vi "SerialRead.vi"() -> ()   [LabVIEW 2013]
uses:
  <vilib>/Analysis/3filter.llb/Filter Passband Type.ctl
  <vilib>/Instr/_visa.llb/VISA Configure Serial Port (Instr).vi
  <vilib>/Analysis/3filter.llb/Butterworth Filter (DBL).vi
  <vilib>/Analysis/NI_AALBase.lvlib
panel:
  in  "?":bool
  out "time":dbl
  in  "high_time":i32
  in  "low_time":i32
  out "diferença":dbl
  out "high_time":dbl format="%#_10g"
  out "low_time":dbl format="%#_10g"
  in  "stop":bool
  in  "high":u32
  in  "low":i32
  in  "Pcell1":u32[](array[numeric])
  in  "Pcell2":u32[](array[numeric])
  in  "Pcell3":u32[](array[numeric])
  in  "Pcell4":u32[](array[numeric])
  in  "cell1":u32[](array[numeric])
  in  "cell2":u32[](array[numeric])
  in  "cell3":u32[](array[numeric])
  in  "cell4":u32[](array[numeric])
  in  "last":u32
  out "time":u32[](graph)
  in  "Tab Control":enum32{"raw data", "filter", "weight"}(tab)
  out "filter_cell2":dbl[](graph) caption="Sine"
  out "filter_cell4":dbl[](graph) caption="Sine"
  out "filter_cell3":dbl[](graph) caption="Sine"
  out "filter_cell1":dbl[](graph) caption="Sine"
  out "peso_cell2":dbl[](graph) caption="Sine"
  out "peso_cell3":dbl[](graph) caption="Sine"
  out "peso_cell4":dbl[](graph) caption="Sine"
  out "peso_cell1":dbl[](graph) caption="Sine"
  out "cell":u8[](array[numeric])
  out "output_int16":i32[](array[numeric])
  out "data":u8[](array[numeric])
  in  "serial_port":refnum<visa-resource-name> caption="Porta Serial"
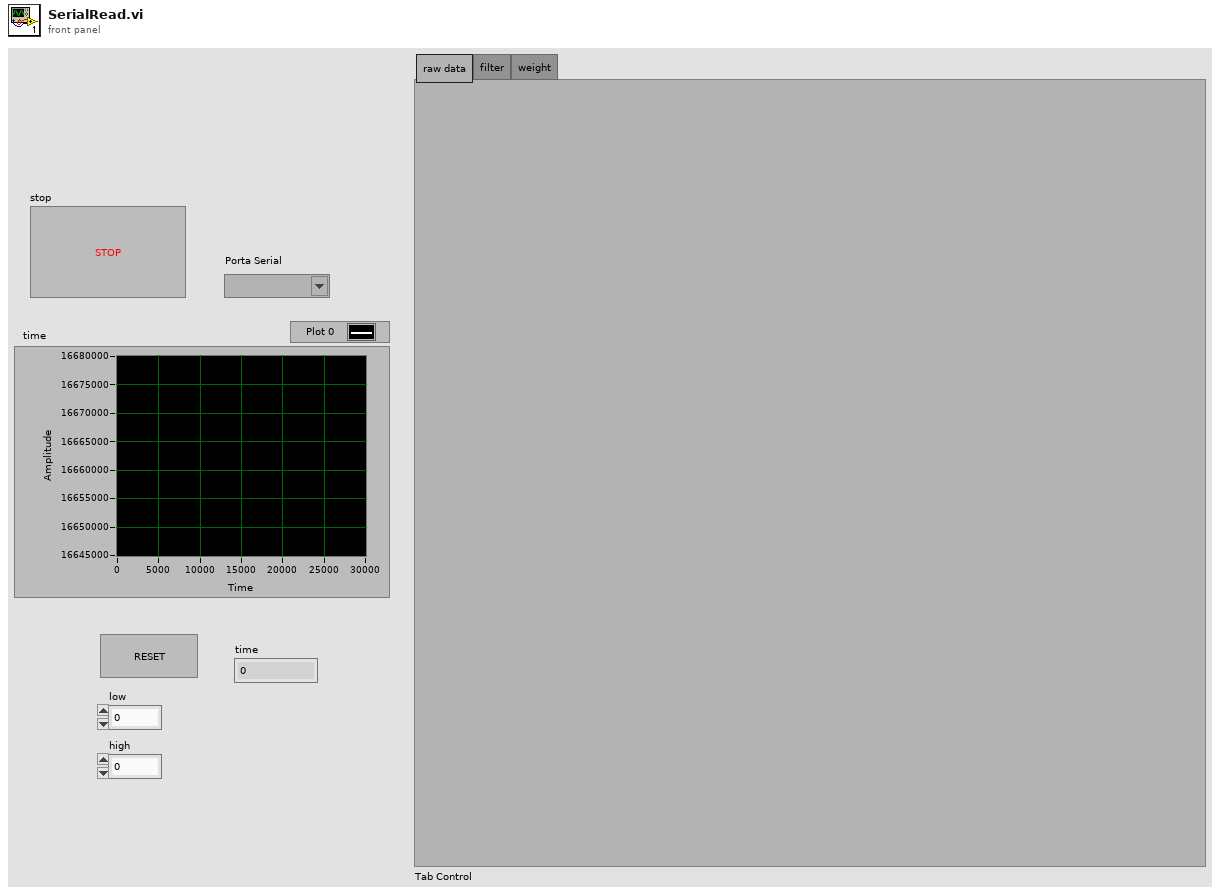
[diagram p1: front panel]
types:
  T1 = typedef "NI_AALBase.lvlib/Filter Passband Type.ctl" = enum32{"Lowpass", "Highpass", "Bandpass", "Bandstop"}
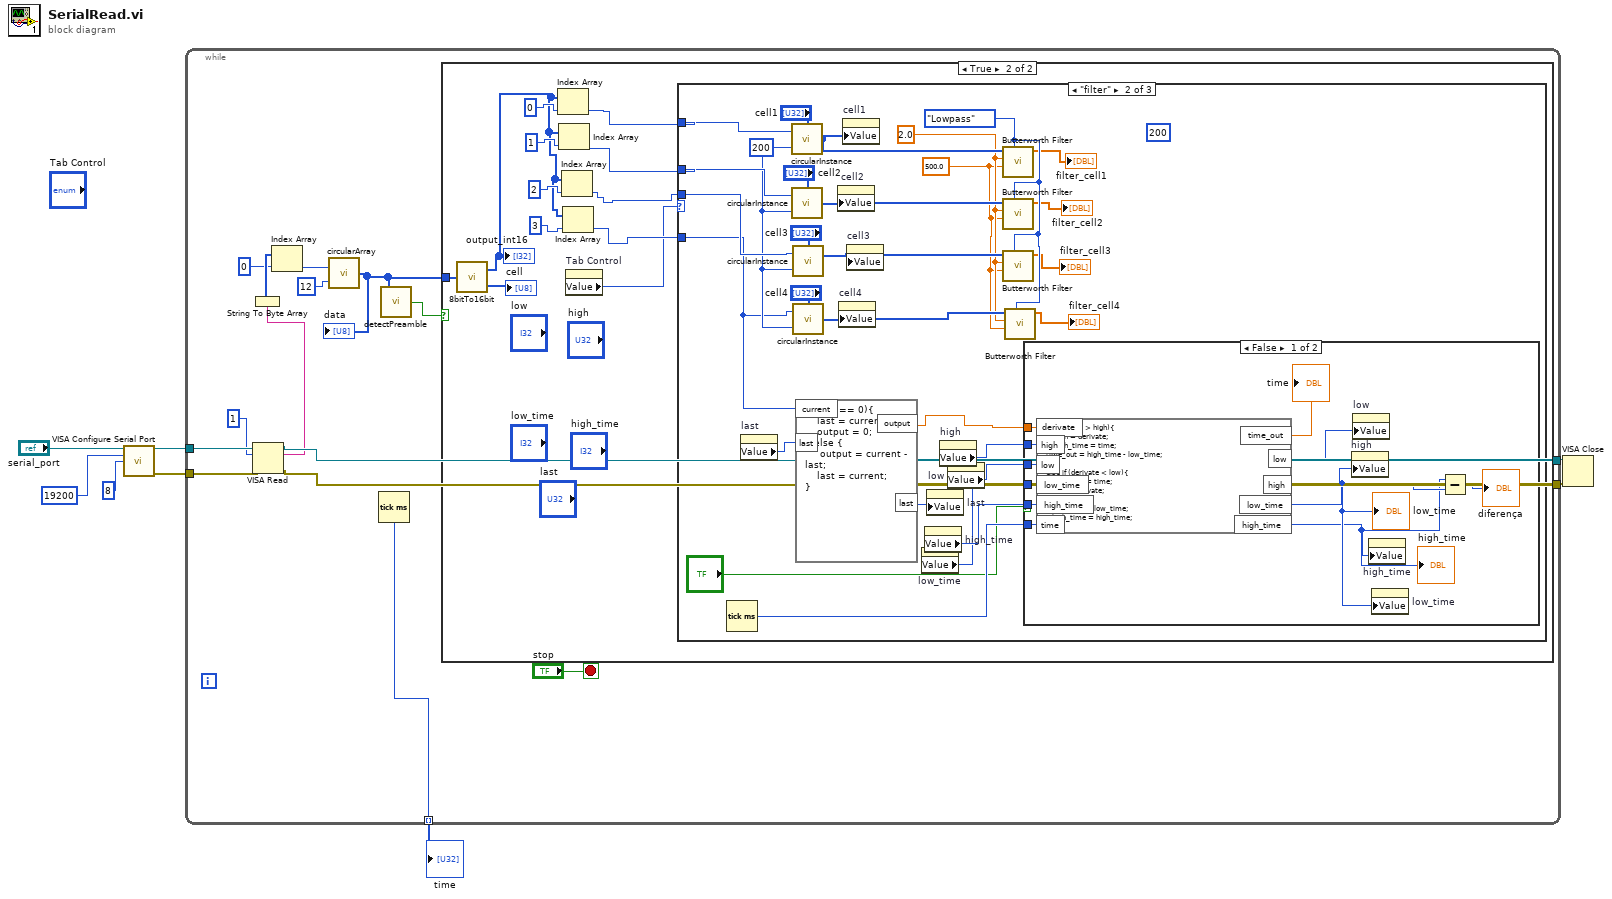
[diagram p0: block diagram]
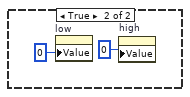
[diagram p4: hidden frame]
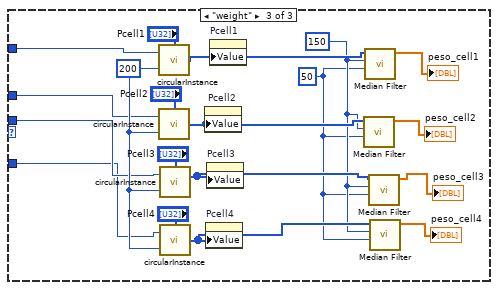
[diagram p5: hidden frame]
diagram:
  n1 = call-poly "VISA Configure Serial Port"("VISA resource name"="serial_port", "baud rate (9600)"=u32 19200, "data bits (8)"=u16 8) -> ("VISA resource name out"=w5:refnum<visa-resource-name>, "error out"=w4:errorcluster)  [unwired: 11 in]
  n2 = while {
    tunnel: w5 -> [w22]
    tunnel: w4 -> [w21]
    tunnel: [w19] -> w2
    tunnel: [w20] -> w3
    tunnel: [w10] -> w1 mode=indexing
    stop <- "stop" stop-if-true
    n3 = VISA Read(VISA resource name=w22, byte count=1, error in (no error)=w21) -> (VISA resource name out=w20:refnum<visa-resource-name>, read buffer=w14:string, error out=w19:errorcluster)  [unwired: 1 out]
    n4 = String To Byte Array(string=w14) -> (unsigned byte array=w17:u8[])
    n5 = Index Array(array=w17, index=0) -> (element=w11:u8)
    n6 = call "circularArray.vi"("max-size"=u8 12, "element"=w11) -> ("dataout"=w12:u8[])
    "data" <- w12
    n7 = Tick Count (ms)() -> (millisecond timer value=w10:u32)
    n8 = call "detectPreamble.vi"("data-in"=w12) -> ("detected"=w9:bool)
    n9 = case shown="True" w9 {
      tunnel: w12 -> [_ w33]
      frame False {
      }
      frame True {
        n10 = call "8bitTo16bit.vi"("input_byte"=w33) -> ("output_int16"=w28:i32[], "cell"=→"cell":u8[])
        "output_int16" <- w28
        n11 = Index Array(array=w28, index=0) -> (element=w24:i32)
        n12 = Index Array(array=w28, index=1) -> (element=w25:i32)
        n13 = Index Array(array=w28, index=2) -> (element=w26:i32)
        n14 = Index Array(array=w28, index=3) -> (element=w27:i32)
        n15 = property on="Tab Control" class="TabCtl (strict)"() -> ("Value"=w23:enum32{"raw data", "filter", "weight"})  [unwired: 2 in, 2 out]
        n16 = case shown="\"filter\"" w23 {
          tunnel: w24 -> [_ w63 w91]
          tunnel: w25 -> [_ w62 w90]
          tunnel: w26 -> [_ w57 w89]
          tunnel: w27 -> [_ w44 w88]
          frame "raw data", Default {
          }
          frame "filter" {
            (unwired) 200
            w52 = 2.0 ("sampling freq: fs")
            w51 = 500.0 ("high cutoff freq: fh")
            w50 = Filter_Passband_Type."Lowpass" ("filter type")
            w46 = i16 200 ("max-size")
            n17 = Tick Count (ms)() -> (millisecond timer value=w37:u32)
            n18 = property on="last" class="DigNum (strict)"() -> ("Value"=w45:u32)  [unwired: 2 in, 2 out]
            n19 = call "circularInstance.vi"("data"="cell1", "max-size"=w46, "element"=w63) -> ("dataout"=w58:u32[])
            n20 = call "circularInstance.vi"("data"="cell2", "max-size"=w46, "element"=w62) -> ("dataout"=w59:u32[])
            n21 = call "circularInstance.vi"("data"="cell3", "max-size"=w46, "element"=w57) -> ("dataout"=w55:u32[])
            n22 = call "circularInstance.vi"("data"="cell4", "max-size"=w46, "element"=w44) -> ("dataout"=w53:u32[])
            n23 = formula code="if (last == 0){\n    last = current;\n    output = 0;\n} else {\n     output = current - last;\n    last = current;\n}"("last"=w45, "current"=w44) -> ("output"=w42:dbl, "last"=w43:u32)
            n24 = property on="cell2" class="Arr (strict)"("Value"=w59) -> ()  [unwired: 2 in, 2 out]
            n25 = property on="cell4" class="Arr (strict)"("Value"=w53) -> ()  [unwired: 2 in, 2 out]
            n26 = property on="cell1" class="Arr (strict)"("Value"=w58) -> ()  [unwired: 2 in, 2 out]
            n27 = property on="cell3" class="Arr (strict)"("Value"=w55) -> ()  [unwired: 2 in, 2 out]
            n28 = property on="low_time" class="DigNum (strict)"() -> ("Value"=w38:i32)  [unwired: 2 in, 2 out]
            n29 = property on="high_time" class="DigNum (strict)"() -> ("Value"=w39:i32)  [unwired: 2 in, 2 out]
            n30 = property on="last" class="DigNum (strict)"("Value"=w43) -> ()  [unwired: 2 in, 2 out]
            n31 = property on="high" class="DigNum (strict)"() -> ("Value"=w41:u32)  [unwired: 2 in, 2 out]
            n32 = property on="low" class="DigNum (strict)"() -> ("Value"=w40:i32)  [unwired: 2 in, 2 out]
            n33 = call-poly <vilib>:"Butterworth Filter.vi"("filter type"=w50, "high cutoff freq: fh"=w51, "sampling freq: fs"=w52, "X"=w58) -> ("Filtered X"=→"filter_cell1":dbl[])  [unwired: 4 in, 1 out]
            n34 = call-poly <vilib>:"Butterworth Filter.vi"("filter type"=w50, "high cutoff freq: fh"=w51, "sampling freq: fs"=w52, "X"=w59) -> ("Filtered X"=→"filter_cell2":dbl[])  [unwired: 4 in, 1 out]
            n35 = call-poly <vilib>:"Butterworth Filter.vi"("filter type"=w50, "high cutoff freq: fh"=w51, "sampling freq: fs"=w52, "X"=w55) -> ("Filtered X"=→"filter_cell3":dbl[])  [unwired: 4 in, 1 out]
            n36 = call-poly <vilib>:"Butterworth Filter.vi"("filter type"=w50, "high cutoff freq: fh"=w51, "sampling freq: fs"=w52, "X"=w53) -> ("Filtered X"=→"filter_cell4":dbl[])  [unwired: 4 in, 1 out]
            n37 = case shown="False" "?" {
              tunnel: w42 -> [w75 _]
              tunnel: w41 -> [w74 _]
              tunnel: w40 -> [w73 _]
              tunnel: w39 -> [w69 _]
              tunnel: w38 -> [w68 _]
              tunnel: w37 -> [w65 _]
              frame False {
                n38 = formula code="if (derivate > high){\n    high = derivate;\n    high_time = time;\ntime_out = high_time - low_time;\n}\nelse if (derivate < low){\n   low_time = time;\n   low = derivate;  \n} else {\n   low_time = low_time;\n   high_time = high_time;\n}"("derivate"=w75, "high"=w74, "low"=w73, "time"=w65, "low_time"=w68, "high_time"=w69) -> ("low"=w72:i32, "high"=w71:u32, "low_time"=w67:i32, "high_time"=w66:i32, "time_out"=→"time":dbl)
                "low_time" <- w67
                "high_time" <- w66
                n39 = property on="high" class="DigNum (strict)"("Value"=w71) -> ()  [unwired: 2 in, 2 out]
                n40 = property on="low" class="DigNum (strict)"("Value"=w72) -> ()  [unwired: 2 in, 2 out]
                n41 = property on="high_time" class="DigNum (strict)"("Value"=w66) -> ()  [unwired: 2 in, 2 out]
                n42 = property on="low_time" class="DigNum (strict)"("Value"=w67) -> ()  [unwired: 2 in, 2 out]
                n43 = Subtract(x=w66, y=w67) -> (x-y=→"diferença":i32)
              }
              frame True {
                n44 = property on="low" class="DigNum (strict)"("Value"=0 ("low")) -> ()  [unwired: 2 in, 2 out]
                n45 = property on="high" class="DigNum (strict)"("Value"=u32 0 ("high")) -> ()  [unwired: 2 in, 2 out]
              }
            }
          }
          frame "weight" {
            w82 = 50 ("left rank")
            w83 = 150 ("left rank")
            w94 = i16 200 ("max-size")
            n46 = call "circularInstance.vi"("data"="Pcell1", "max-size"=w94, "element"=w91) -> ("dataout"=w87:u32[])
            n47 = call "circularInstance.vi"("data"="Pcell2", "max-size"=w94, "element"=w90) -> ("dataout"=w86:u32[])
            n48 = call "circularInstance.vi"("data"="Pcell3", "max-size"=w94, "element"=w89) -> ("dataout"=w85:u32[])
            n49 = call "circularInstance.vi"("data"="Pcell4", "max-size"=w94, "element"=w88) -> ("dataout"=w84:u32[])
            n50 = property on="Pcell2" class="Arr (strict)"("Value"=w86) -> ()  [unwired: 2 in, 2 out]
            n51 = property on="Pcell4" class="Arr (strict)"("Value"=w84) -> ()  [unwired: 2 in, 2 out]
            n52 = property on="Pcell3" class="Arr (strict)"("Value"=w85) -> ()  [unwired: 2 in, 2 out]
            n53 = property on="Pcell1" class="Arr (strict)"("Value"=w87) -> ()  [unwired: 2 in, 2 out]
            n54 = call <vilib>:"Median Filter.vi"("right rank"=w82, "left rank"=w83, "X"=w86) -> ("Filtered X"=→"peso_cell2":dbl[])  [unwired: 7 in, 1 out]
            n55 = call <vilib>:"Median Filter.vi"("right rank"=w82, "left rank"=w83, "X"=w87) -> ("Filtered X"=→"peso_cell1":dbl[])  [unwired: 7 in, 1 out]
            n56 = call <vilib>:"Median Filter.vi"("right rank"=w82, "left rank"=w83, "X"=w85) -> ("Filtered X"=→"peso_cell3":dbl[])  [unwired: 7 in, 1 out]
            n57 = call <vilib>:"Median Filter.vi"("right rank"=w82, "left rank"=w83, "X"=w84) -> ("Filtered X"=→"peso_cell4":dbl[])  [unwired: 7 in, 1 out]
          }
        }
      }
    }
  }
  "time" <- w1
  n58 = VISA Close(VISA resource name=w3, error in (no error)=w2) -> ()  [unwired: 1 out]
